vi "ReInit_TCP.vi"(8 "error in (no error)":errorcluster, 11 "Queue in":refnum<queue>) -> (0 "error out":errorcluster)   [LabVIEW 2021]
doc: "If an error occurs while initializing or while reading, close the connection and start again."
uses:
  Controls/Enums/TCP_Loop_Enum.ctl
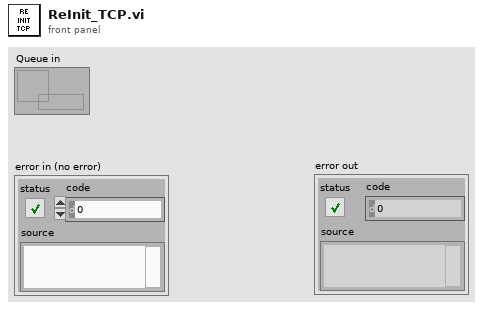
[diagram p1: front panel]
types:
  T1 = typedef "TCP_Loop_Enum.ctl" = enum16{"TCP_Init", "TCP_Read", "TCP_Write", "TCP_Close"}
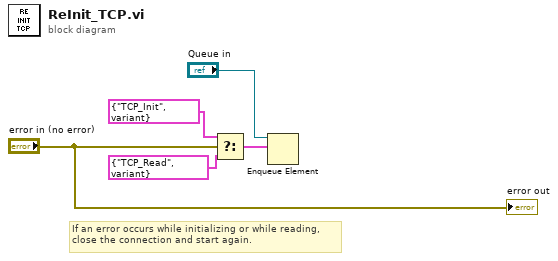
[diagram p0: block diagram]
diagram:
  # "If an error occurs while initializing or while reading,\nclose the connection and start again."
  n1 = Select(t=cluster{T1, variant} {enum."TCP_Init", variant}, s="error in (no error)", f=cluster{T1, variant} {enum."TCP_Read", variant}) -> (s? t:f=w3:cluster{T1, variant})
  n2 = Enqueue Element(queue="Queue in", element=w3) -> ()  [unwired: 2 in, 3 out]
  "error out" <- "error in (no error)"
